vi "test Loopback BC to RT with Start Stop and Status.vi"(8 "error in":errorcluster, 11 "TestCase in":refnum<class "Loopback.lvclass">) -> (0 "error out":errorcluster, 3 "TestCase out":refnum<class "Loopback.lvclass">)   [LabVIEW 2020, in "Loopback.lvclass"]
uses:
  Loopback.lvclass
  C:/dev/niveristand-custom-device-testing-tools/VeriStandTestCase/VeriStandTestCase.lvclass
  <vilib>/numeric/Random Number (Range) U64.vi
  485b7c2b-8320-4722-9ec7-d01f27c65546.vi
  b08989c6-5f8b-4abd-9880-ddf65696a96d.vi
  632f36f1-4b6f-4095-917c-563c19b80c3a.vi
  c8f491d9-e213-4f8e-8b18-a73afe23b1be.vi
  0f9dda61-2c21-4955-8588-a8fc95227647.vi
  33c3b3d1-f053-43c7-bbe8-20c4ad88f1fe.vi
  757b3fb2-d48b-4fbb-8961-a38cd8e327a9.vi
  ff2cfcab-6673-4a18-a151-e28207f633c9.vi
  <vilib>/numeric/sub_Random U32.vi
  <vilib>/NI VeriStand/Execution/Workspace/NI VeriStand - Set Multiple Channel Values.vi
  <vilib>/NI VeriStand/Execution/Workspace/NI VeriStand - Get Multiple Channel Values.vi
  <vilib>/NI VeriStand/Execution/Workspace/NI VeriStand - Set Single Channel Value.vi
  <vilib>/addons/_JKI Toolkits/VI Tester/TestCase.llb/TestCase.lvclass
  <vilib>/NI VeriStand/Execution/Workspace/NI_VS Workspace ExecutionAPI.lvlib
  C:/Program Files (x86)/National Instruments/LabVIEW 2020/vi.lib/addons/_JKI Toolkits/VI Tester/TestCase.llb/TestCase.lvclass
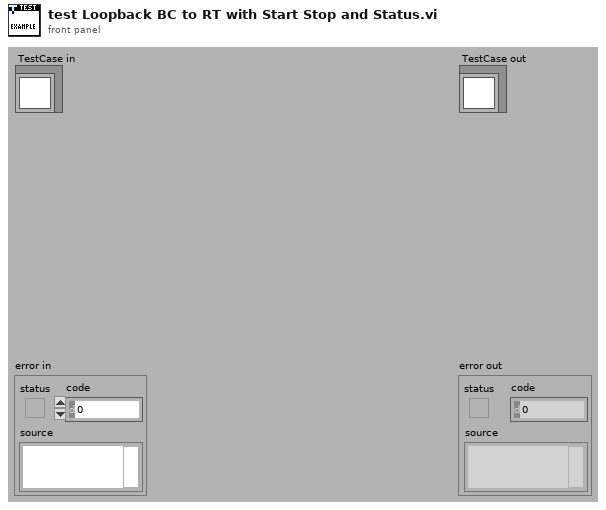
[diagram p1: front panel]
types:
  T1 = typedef "NI_VS Workspace ExecutionAPI.lvlib/WorkspaceAPI.ctl" = refnum<k24>
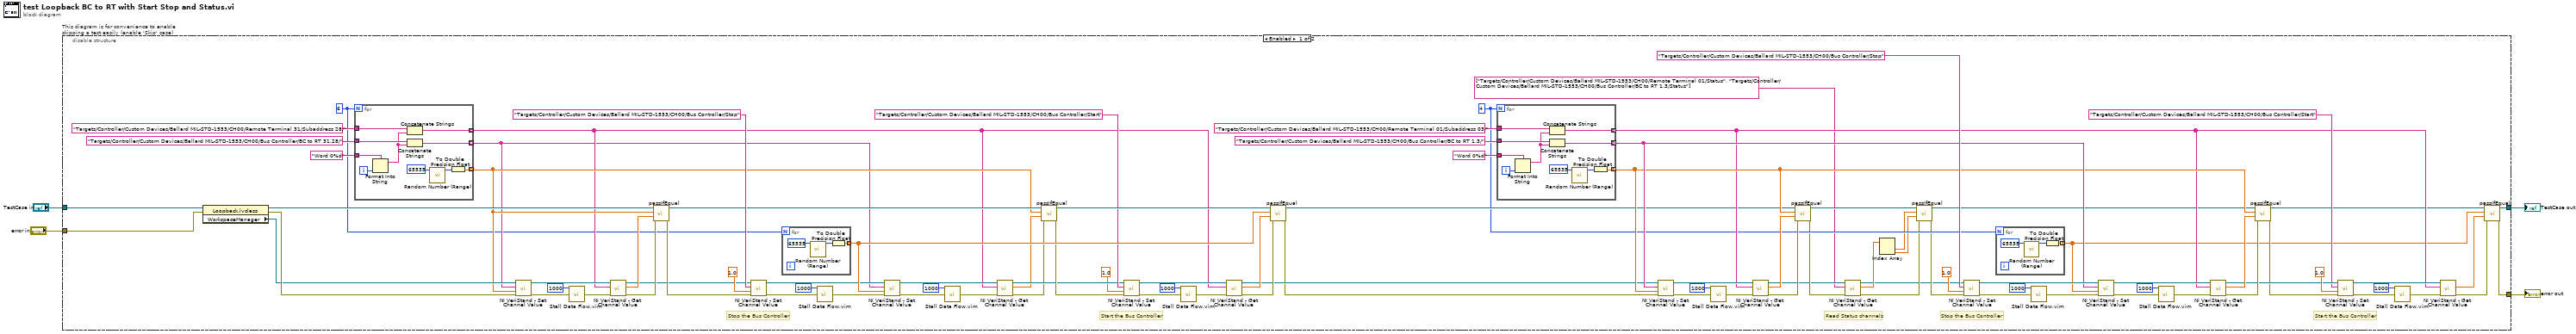
[diagram p0: block diagram]
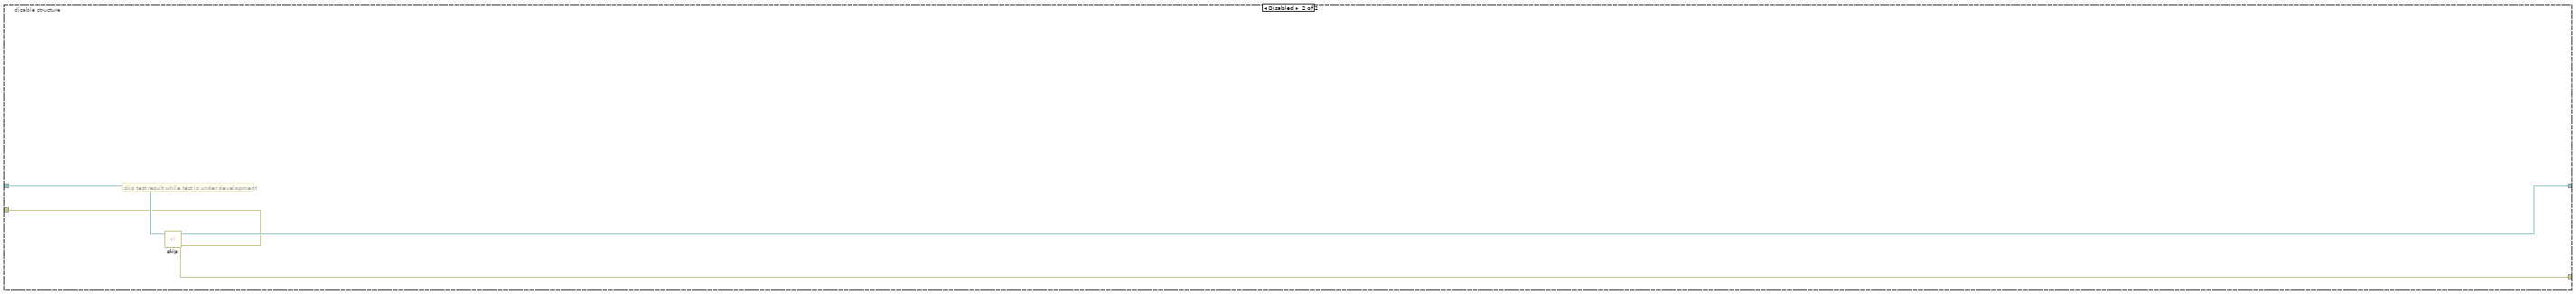
[diagram p2: hidden frame]
diagram:
  n1 = disable-structure "This diagram is for convenience to enable skipping a test easily (enable 'Skip' case)" shown="Enabled" {
    disable-tunnel: "TestCase in" -> [w93 w132]
    disable-tunnel: [w17 w130] -> w1
    disable-tunnel: [w16 w131] -> w3
    disable-tunnel: "error in" -> [w90 w129]
    frame Enabled {
      w18 = 4
      w19 = 6
      # "Read Status channels"
      # "Start the Bus Controller"
      # "Stop the Bus Controller"
      # "Start the Bus Controller"
      # "Stop the Bus Controller"
      n2 = property class="Loopback.lvclass"(reference=w93, error in=w90) -> (reference out=w102:refnum<class "Loopback.lvclass">, error out=w97:errorcluster, "WorkspaceManager"=w95:T1)
      n3 = for {
        N: w19 -> [_]
        tunnel: "Targets/Controller/Custom Devices/Ballard MIL-STD-1553/CH00/Bus Controller/BC to RT 31.28/" ("Channel") -> [w124]
        tunnel: [w125] -> w21 mode=indexing
        tunnel: "Targets/Controller/Custom Devices/Ballard MIL-STD-1553/CH00/Remote Terminal 31/Subaddress 28/" ("Channel") -> [w123]
        tunnel: [w122] -> w22 mode=indexing
        tunnel: "Word 0%d" -> [w120]
        tunnel: [w116] -> w23 mode=indexing
        i -> [w121]
        n4 = Format Into String(format string=w120, w121) -> (resulting string=w119:string)  [unwired: 2 in, 1 out]
        n5 = Concatenate Strings(w123, w119) -> (w122:string)
        n6 = Concatenate Strings(w124, w119) -> (w125:string)
        n7 = call-poly <vilib>:"Random Number (Range).vi"("upper bound (100)"=u64 65535) -> ("number"=w118:u64)  [unwired: 10 in]
        n8 = To Double Precision Float(number=w118) -> (double precision float=w116:dbl)
      }
      n9 = call-poly <vilib>:"NI VeriStand - Set Channel Value.vi"("error in (no error)"=w97, "Values"=w23, "Channels"=w21, "WorkspaceManager in"=w95) -> ("error out"=w99:errorcluster, "WorkspaceManager out"=w101:T1)  [unwired: 6 in]
      n10 = call "Stall Data Flow.vim"("value in"=w99, "milliseconds to wait"=u32 1000) -> ("value out"=w100:errorcluster)  [unwired: 1 out]
      n11 = call-poly <vilib>:"NI VeriStand - Get Channel Value.vi"("error in (no error)"=w100, "Channels"=w22, "WorkspaceManager in"=w101) -> ("error out"=w96:errorcluster, "Values"=w94:dbl[], "WorkspaceManager out"=w25:T1)  [unwired: 6 in]
      n12 = call-dynamic "passIfEqual.vi"("error in (no error)"=w96, "y"=w94, "x"=w23, "TestCase in"=w102) -> ("error out"=w26:errorcluster, "TestCase out"=w24:refnum<class "Loopback.lvclass">)  [unwired: 6 in]
      n13 = call-poly <vilib>:"NI VeriStand - Set Channel Value.vi"("error in (no error)"=w26, "Value"=1.0, "Channel"="Targets/Controller/Custom Devices/Ballard MIL-STD-1553/CH00/Bus Controller/Stop", "WorkspaceManager in"=w25) -> ("error out"=w51:errorcluster, "WorkspaceManager out"=w31:T1)  [unwired: 6 in]
      n14 = for {
        N: w19 -> [_]
        tunnel: [w113] -> w45 mode=indexing
        n15 = call-poly <vilib>:"Random Number (Range).vi"("upper bound (100)"=u64 65535) -> ("number"=w114:u64)  [unwired: 10 in]
        n16 = To Double Precision Float(number=w114) -> (double precision float=w113:dbl)
      }
      n17 = call "Stall Data Flow.vim"("value in"=w51, "milliseconds to wait"=u32 1000) -> ("value out"=w52:errorcluster)  [unwired: 1 out]
      n18 = call-poly <vilib>:"NI VeriStand - Set Channel Value.vi"("error in (no error)"=w52, "Values"=w45, "Channels"=w21, "WorkspaceManager in"=w31) -> ("error out"=w47:errorcluster, "WorkspaceManager out"=w32:T1)  [unwired: 6 in]
      n19 = call "Stall Data Flow.vim"("value in"=w47, "milliseconds to wait"=u32 1000) -> ("value out"=w48:errorcluster)  [unwired: 1 out]
      n20 = call-poly <vilib>:"NI VeriStand - Get Channel Value.vi"("error in (no error)"=w48, "Channels"=w22, "WorkspaceManager in"=w32) -> ("error out"=w33:errorcluster, "Values"=w34:dbl[], "WorkspaceManager out"=w36:T1)  [unwired: 6 in]
      n21 = call-dynamic "passIfEqual.vi"("error in (no error)"=w33, "y"=w34, "x"=w23, "TestCase in"=w24) -> ("error out"=w40:errorcluster, "TestCase out"=w49:refnum<class "Loopback.lvclass">)  [unwired: 6 in]
      n22 = call-poly <vilib>:"NI VeriStand - Set Channel Value.vi"("error in (no error)"=w40, "Value"=1.0, "Channel"="Targets/Controller/Custom Devices/Ballard MIL-STD-1553/CH00/Bus Controller/Start", "WorkspaceManager in"=w36) -> ("error out"=w39:errorcluster, "WorkspaceManager out"=w44:T1)  [unwired: 6 in]
      n23 = call "Stall Data Flow.vim"("value in"=w39, "milliseconds to wait"=u32 1000) -> ("value out"=w43:errorcluster)  [unwired: 1 out]
      n24 = call-poly <vilib>:"NI VeriStand - Get Channel Value.vi"("error in (no error)"=w43, "Channels"=w22, "WorkspaceManager in"=w44) -> ("error out"=w42:errorcluster, "Values"=w41:dbl[], "WorkspaceManager out"=w27:T1)  [unwired: 6 in]
      n25 = call-dynamic "passIfEqual.vi"("error in (no error)"=w42, "y"=w41, "x"=w45, "TestCase in"=w49) -> ("error out"=w20:errorcluster, "TestCase out"=w28:refnum<class "Loopback.lvclass">)  [unwired: 6 in]
      n26 = for {
        N: w18 -> [_]
        tunnel: "Targets/Controller/Custom Devices/Ballard MIL-STD-1553/CH00/Bus Controller/BC to RT 1.3/" ("Channel") -> [w111]
        tunnel: [w112] -> w76 mode=indexing
        tunnel: "Targets/Controller/Custom Devices/Ballard MIL-STD-1553/CH00/Remote Terminal 01/Subaddress 03/" ("Channel") -> [w110]
        tunnel: [w109] -> w61 mode=indexing
        tunnel: "Word 0%d" -> [w107]
        tunnel: [w103] -> w72 mode=indexing
        i -> [w108]
        n27 = Format Into String(format string=w107, w108) -> (resulting string=w106:string)  [unwired: 2 in, 1 out]
        n28 = Concatenate Strings(w110, w106) -> (w109:string)
        n29 = Concatenate Strings(w111, w106) -> (w112:string)
        n30 = call-poly <vilib>:"Random Number (Range).vi"("upper bound (100)"=u64 65535) -> ("number"=w105:u64)  [unwired: 10 in]
        n31 = To Double Precision Float(number=w105) -> (double precision float=w103:dbl)
      }
      n32 = call-poly <vilib>:"NI VeriStand - Set Channel Value.vi"("error in (no error)"=w20, "Values"=w72, "Channels"=w76, "WorkspaceManager in"=w27) -> ("error out"=w82:errorcluster, "WorkspaceManager out"=w80:T1)  [unwired: 6 in]
      n33 = call "Stall Data Flow.vim"("value in"=w82, "milliseconds to wait"=u32 1000) -> ("value out"=w81:errorcluster)  [unwired: 1 out]
      n34 = call-poly <vilib>:"NI VeriStand - Get Channel Value.vi"("error in (no error)"=w81, "Channels"=w61, "WorkspaceManager in"=w80) -> ("error out"=w84:errorcluster, "Values"=w85:dbl[], "WorkspaceManager out"=w13:T1)  [unwired: 6 in]
      n35 = call-dynamic "passIfEqual.vi"("error in (no error)"=w84, "y"=w85, "x"=w72, "TestCase in"=w28) -> ("error out"=w14:errorcluster, "TestCase out"=w12:refnum<class "Loopback.lvclass">)  [unwired: 6 in]
      n36 = call-poly <vilib>:"NI VeriStand - Get Channel Value.vi"("error in (no error)"=w14, "Channels"=string[] ["Targets/Controller/Custom Devices/Ballard MIL-STD-1553/CH00/Remote Terminal 01/Status", "Targets/Controller/Custom Devices/Ballard MIL-STD-1553/CH00/Bus Controller/BC to RT 1.3/Status"], "WorkspaceManager in"=w13) -> ("error out"=w15:errorcluster, "Values"=w11:dbl[], "WorkspaceManager out"=w6:T1)  [unwired: 6 in]
      n37 = Index Array(array=w11) -> (element #1=w10:dbl, element #2=w9:dbl)  [unwired: 2 in]
      n38 = call-dynamic "passIfEqual.vi"("error in (no error)"=w15, "y"=w9, "x"=w10, "TestCase in"=w12) -> ("error out"=w8:errorcluster, "TestCase out"=w7:refnum<class "Loopback.lvclass">)  [unwired: 6 in]
      n39 = call-poly <vilib>:"NI VeriStand - Set Channel Value.vi"("error in (no error)"=w8, "Value"=1.0, "Channel"="Targets/Controller/Custom Devices/Ballard MIL-STD-1553/CH00/Bus Controller/Stop", "WorkspaceManager in"=w6) -> ("error out"=w54:errorcluster, "WorkspaceManager out"=w77:T1)  [unwired: 6 in]
      n40 = for {
        N: w18 -> [_]
        tunnel: [w126] -> w60 mode=indexing
        n41 = call-poly <vilib>:"Random Number (Range).vi"("upper bound (100)"=u64 65535) -> ("number"=w127:u64)  [unwired: 10 in]
        n42 = To Double Precision Float(number=w127) -> (double precision float=w126:dbl)
      }
      n43 = call "Stall Data Flow.vim"("value in"=w54, "milliseconds to wait"=u32 1000) -> ("value out"=w53:errorcluster)  [unwired: 1 out]
      n44 = call-poly <vilib>:"NI VeriStand - Set Channel Value.vi"("error in (no error)"=w53, "Values"=w60, "Channels"=w76, "WorkspaceManager in"=w77) -> ("error out"=w58:errorcluster, "WorkspaceManager out"=w75:T1)  [unwired: 6 in]
      n45 = call "Stall Data Flow.vim"("value in"=w58, "milliseconds to wait"=u32 1000) -> ("value out"=w57:errorcluster)  [unwired: 1 out]
      n46 = call-poly <vilib>:"NI VeriStand - Get Channel Value.vi"("error in (no error)"=w57, "Channels"=w61, "WorkspaceManager in"=w75) -> ("error out"=w74:errorcluster, "Values"=w73:dbl[], "WorkspaceManager out"=w70:T1)  [unwired: 6 in]
      n47 = call-dynamic "passIfEqual.vi"("error in (no error)"=w74, "y"=w73, "x"=w72, "TestCase in"=w7) -> ("error out"=w66:errorcluster, "TestCase out"=w56:refnum<class "Loopback.lvclass">)  [unwired: 6 in]
      n48 = call-poly <vilib>:"NI VeriStand - Set Channel Value.vi"("error in (no error)"=w66, "Value"=1.0, "Channel"="Targets/Controller/Custom Devices/Ballard MIL-STD-1553/CH00/Bus Controller/Start", "WorkspaceManager in"=w70) -> ("error out"=w67:errorcluster, "WorkspaceManager out"=w62:T1)  [unwired: 6 in]
      n49 = call "Stall Data Flow.vim"("value in"=w67, "milliseconds to wait"=u32 1000) -> ("value out"=w63:errorcluster)  [unwired: 1 out]
      n50 = call-poly <vilib>:"NI VeriStand - Get Channel Value.vi"("error in (no error)"=w63, "Channels"=w61, "WorkspaceManager in"=w62) -> ("error out"=w64:errorcluster, "Values"=w65:dbl[])  [unwired: 6 in, 1 out]
      n51 = call-dynamic "passIfEqual.vi"("error in (no error)"=w64, "y"=w65, "x"=w60, "TestCase in"=w56) -> ("error out"=w16:errorcluster, "TestCase out"=w17:refnum<class "Loopback.lvclass">)  [unwired: 6 in]
    }
    frame Disabled {
      # "skip test result while test is under development"
      n52 = call <vilib>:"skip.vi"("error in (no error)"=w129, "TestCase in"=w132) -> ("error out"=w131:errorcluster, "TestCase out"=w130:refnum<class "Loopback.lvclass">)  [unwired: 8 in]
    }
  }
  "error out" <- w3
  "TestCase out" <- w1
